vi "Ejemplo_BucleWhile.vi"() -> ()   [LabVIEW 2022 SP3]
panel:
  in  "stop":bool
  out "No. Iteraciones":i32
  out "Número aleatorio":dbl
  in  "Seleccione un \nnúmero entre 0 y 10":dbl
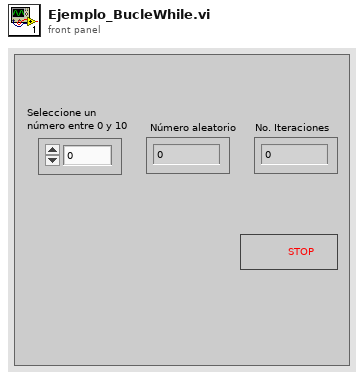
[diagram p1: front panel]
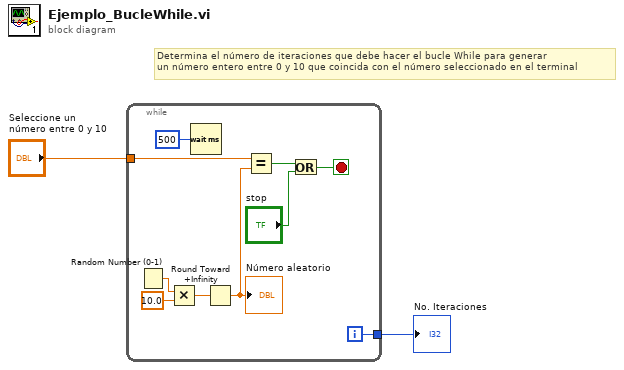
[diagram p0: block diagram]
diagram:
  # "Determina el número de iteraciones que debe hacer el bucle While para generar\nun número entero entre 0 y 10 que coincida con el número seleccionado en el terminal"
  n1 = while {
    tunnel: "Seleccione un \nnúmero entre 0 y 10" -> [w8]
    tunnel: [w6] -> w1
    i -> [w6]
    stop <- w3 stop-if-true
    n2 = Random Number (0-1)() -> (number: 0 to 1=w12:dbl)
    n3 = Multiply(x=w12, y=10.0) -> (x*y=w10:dbl)
    n4 = Wait (ms)(milliseconds to wait=u32 500) -> ()  [unwired: 1 out]
    n5 = Round Toward +Infinity(x=w10) -> (ceil(x): smallest int >= x=w7:dbl)
    "Número aleatorio" <- w7
    n6 = Equal?(x=w8, y=w7) -> (x = y?=w4:bool)
    n7 = Or(x=w4, y="stop") -> (x .or. y?=w3:bool)
  }
  "No. Iteraciones" <- w1
